vi "Version 1_Initialize.vi"(8 "error in (no error)":errorcluster, 11 "VISA Sesson in":refnum<visa-resource-name>) -> (0 "error out":errorcluster, 3 "VISA Session out":refnum<visa-resource-name>)   [LabVIEW 2014]
uses:
  <vilib>/Instr/_visa.llb/VISA Open Access Mode.ctl
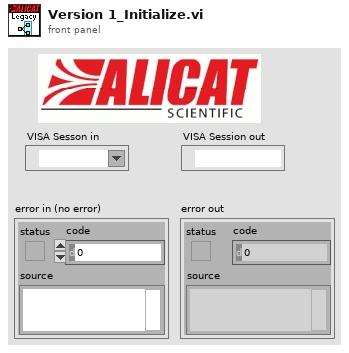
[diagram p1: front panel]
types:
  T1 = typedef "VISA Open Access Mode.ctl" = u32
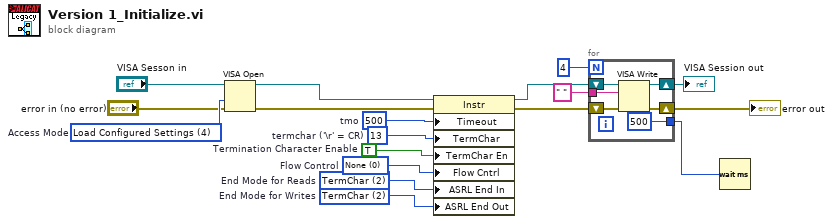
[diagram p0: block diagram]
diagram:
  w10 = u32 500  # tmo
  w13 = T1 4 items=["VISA Defaults"=0, "Exclusive Lock"=1, "Load Configured Settings"=4]  # Access Mode
  w14 = u16 2 items=["None", "Last Bit", "TermChar", "Break"]  # End Mode for Writes
  w15 = u16 2 items=["None", "Last Bit", "TermChar"]  # End Mode for Reads
  w16 = u16 0 items=["None", "XON/XOFF", "RTS/CTS", "XON/XOFF & RTS/CTS", "DTR/DSR", "XON/XOFF & DTR/DSR"]  # Flow Control
  w17 = TRUE  # Termination Character Enable
  w18 = u8 13  # termchar ('\r' = CR)
  n1 = VISA Open(access mode=w13, error in (no error)="error in (no error)", VISA resource name="VISA Sesson in") -> (VISA resource name=w2:refnum<visa-resource-name>, error out=w12:errorcluster)  [unwired: 2 in]
  n2 = property class="Instr"(reference=w2, error in=w12, "Timeout"=w10, "TermChar"=w18, "TermChar En"=w17, "Flow Cntrl"=w16, "ASRL End In"=w15, "ASRL End Out"=w14) -> (reference out=w7:refnum<visa-resource-name>, error out=w9:errorcluster)
  n3 = for {
    N: 4 -> [_]
    tunnel: " " -> [w20]
    shift-right: [w21] -> w1
    shift-left: w7 -> [w22]
    shift-right: [w23] -> w8
    shift-left: w9 -> [w24]
    tunnel: [u32 500 ("milliseconds to wait")] -> w5
    n4 = VISA Write(VISA resource name=w22, write buffer=w20, error in (no error)=w24) -> (VISA resource name out=w21:refnum<visa-resource-name>, error out=w23:errorcluster)  [unwired: 1 out]
  }
  "error out" <- w8
  "VISA Session out" <- w1
  n5 = Wait (ms)(milliseconds to wait=w5) -> ()  [unwired: 1 out]
